vi "Init.vi"(8 "error in (no error)":errorcluster, 10 "isAddrLow(76)":bool) -> (0 "error out":errorcluster, 3 "BME680 out":refnum<class "BME680.lvclass">)   [LabVIEW 2022 SP3, in "BME680.lvlib" / "BME680.lvclass"]
uses:
  BME680.lvclass
  BME680.lvclass/BME680.ctl
  <vilib>/MakerHub/LINX/LMH-LINX.lvlib
  <vilib>/MakerHub/LINX/Public/Utilities/Open Local.vi
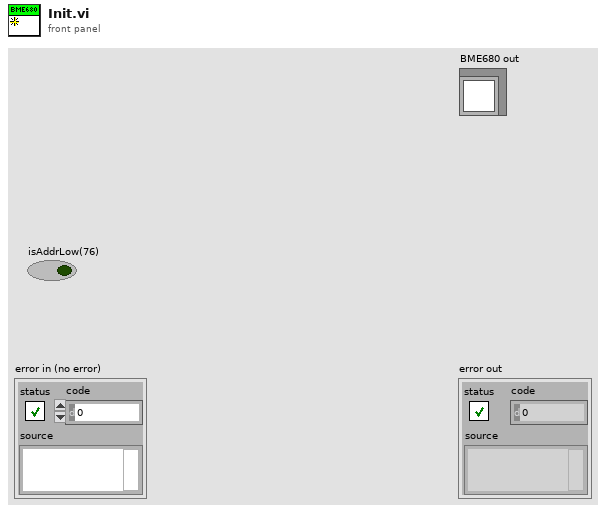
[diagram p1: front panel]
types:
  T1 = typedef "LMH-LINX.lvlib/LINX Ref.ctl" = cluster{"IO":T2, "Interface":T3, "LINX Device Config":T4}
  T2 = typedef "LMH-LINX.lvlib/Platform.ctl" = enum16{"Remote", "Local"}
  T3 = typedef "LMH-LINX.lvlib/Interface.ctl" = enum16{"Serial", "TCP"}
  T4 = typedef "LMH-LINX.lvlib/Device.lvlib/LINX Device Config.ctl" = cluster{"Interface":T3, "COM Port":refnum<visa-resource-name>, "TCP Configuration":T5, "Device Family":u8, "Device ID":u8, "Device Name":string, "TCP Ref":refnum<k5>, "Channels":T6}
  T5 = typedef "LMH-LINX.lvlib/Device.lvlib/TCP Config.ctl" = cluster{"IP Address":string, "Port":u16}
  T6 = typedef "LMH-LINX.lvlib/Channels.ctl" = cluster{"DI":u8[], "DO":u8[], "AI":u8[], "AO":u8[], "PWM":u8[], "QE":u8[], "UART":u8[], "I2C 2":u8[], "SPI":u8[], "CAN":u8[], "Servo":u8[], "AI Ref (V)":dbl, "AI Resolution (Bits)":u8, "AO Ref (V)":dbl, "AO Resolution (Bits)":u8}
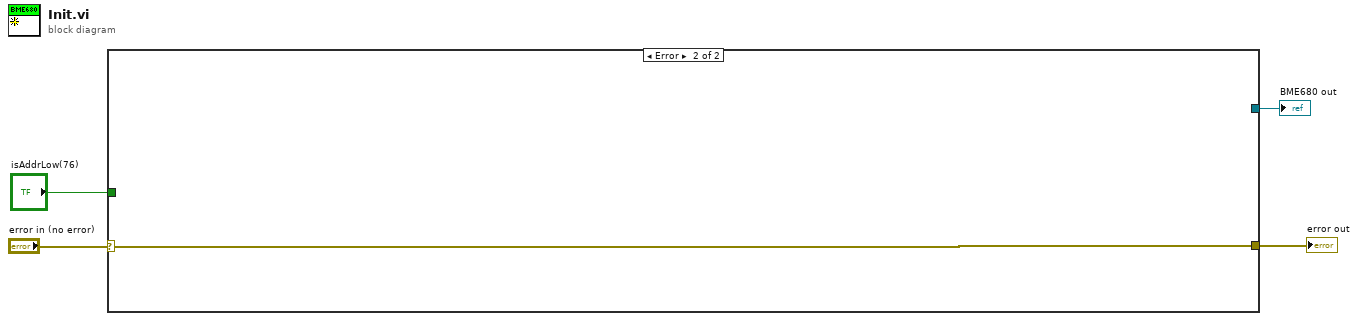
[diagram p0: block diagram]
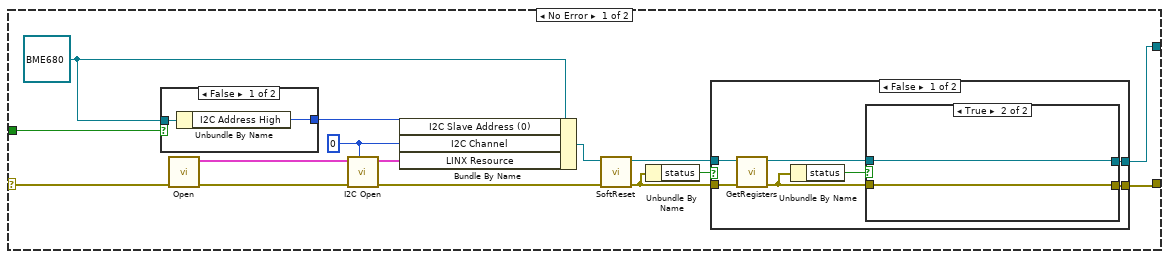
[diagram p2: hidden frame]
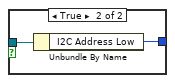
[diagram p3: hidden frame]
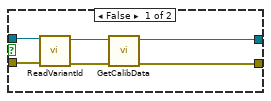
[diagram p4: hidden frame]
diagram:
  n1 = case shown="Error" "error in (no error)" {
    selector: "error in (no error)" -> [w17 w41]
    tunnel: [w5 w41] -> w3
    tunnel: [w18 _] -> w2
    tunnel: "isAddrLow(76)" -> [w16 _]
    frame No Error {
      w8 = u8 0 ("Linx I2C.I2C Channel")
      w15 = refnum<class "BME680.lvclass"> refnum ("BME680 in")
      n2 = case shown="False" w16 {
        tunnel: w15 -> [w21 w23]
        tunnel: [w20 w22] -> w14
        frame False {
          n3 = Unbundle By Name(w21) -> ("I2C Address High"=w20:u8)
        }
        frame True {
          n4 = Unbundle By Name(w23) -> ("I2C Address Low"=w22:u8)
        }
      }
      n5 = call-poly <vilib>:"Open.vi"("Error In"=w17) -> ("Error Out"=w12:errorcluster, "LINX Resource"=w11:T1)  [unwired: 8 in, 1 out]
      n6 = call <vilib>:"I2C Open.vi"("I2C Channel (0)"=w8, "Error In"=w12, "LINX Resource"=w11) -> ("Error Out"=w10:errorcluster, "LINX Resource"=w9:T1)  [unwired: 7 in]
      n7 = Bundle By Name(cluster=w15, "I2C Slave Address (0)"=w14, "I2C Channel"=w8, "LINX Resource"=w9) -> (w13:refnum<class "BME680.lvclass">)
      n8 = call-dynamic "SoftReset.vi"("error in (no error)"=w10, "BME680 in"=w13) -> ("error out"=w7:errorcluster, "BME680 out"=w19:refnum<class "BME680.lvclass">)  [unwired: 8 in]
      n9 = Unbundle By Name(w7) -> ("status"=w6:bool)
      n10 = case shown="False" w6 {
        tunnel: w19 -> [w30 w39]
        tunnel: w7 -> [w29 w40]
        tunnel: [w28 w39] -> w18
        tunnel: [w24 w40] -> w5
        frame False {
          n11 = call-dynamic "GetRegisters.vi"("error in (no error)"=w29, "BME680 in"=w30) -> ("error out"=w27:errorcluster, "BME680 out"=w26:refnum<class "BME680.lvclass">)  [unwired: 7 in, 1 out]
          n12 = Unbundle By Name(w27) -> ("status"=w25:bool)
          n13 = case shown="True" w25 {
            tunnel: w27 -> [w36 w37]
            tunnel: [w34 w38] -> w28
            tunnel: w26 -> [w33 w38]
            tunnel: [w31 w37] -> w24
            frame False {
              n14 = call "ReadVariantId.vi"("error in (no error)"=w36, "BME68x in"=w33) -> ("error out"=w35:errorcluster, "BME68x out"=w32:refnum<class "BME680.lvclass">)  [unwired: 8 in]
              n15 = call "GetCalibData.vi"("error in (no error)"=w35, "BME68x in"=w32) -> ("error out"=w31:errorcluster, "BME68x out"=w34:refnum<class "BME680.lvclass">)  [unwired: 8 in]
            }
            frame True {
            }
          }
        }
        frame True {
        }
      }
    }
    frame Error {
    }
  }
  "error out" <- w3
  "BME680 out" <- w2
